vi "Galvos.vi"() -> ()   [LabVIEW 2014]
uses:
  <vilib>/Analysis/1siggen.llb/Ramp Pattern by Samples.vi
  <vilib>/Analysis/NI_AALBase.lvlib
panel:
  in  "Relax":dbl=10.0 format="%0.2p"
  in  "FOV /V":dbl=10.0 format="%0.2p"
  in  "Samples /s":dbl=10.0 format="%0.2p"
  in  "Exposure":dbl=10.0 format="%0.2p"
  out "XY Galvo":dbl[](graph)
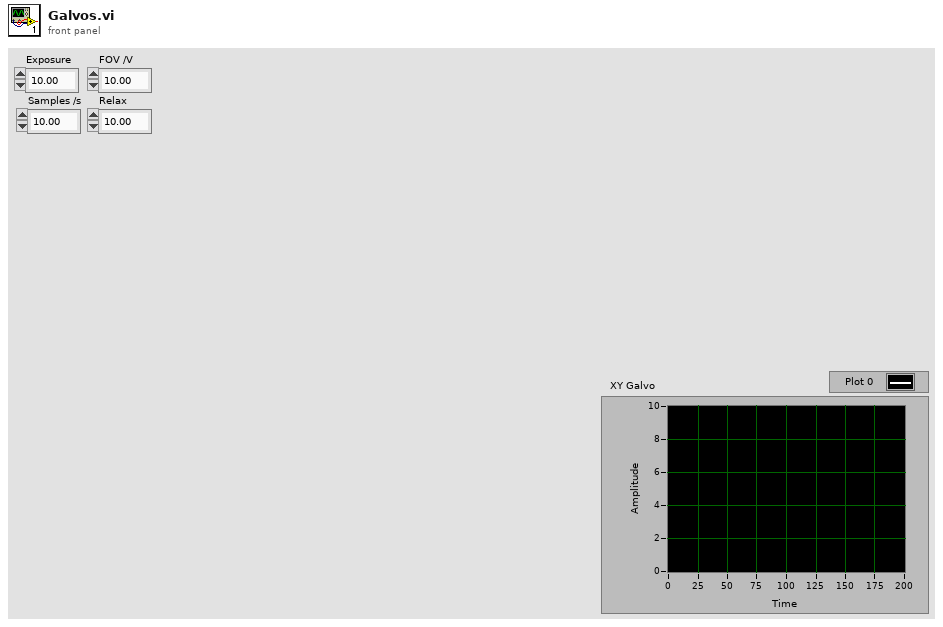
[diagram p1: front panel]
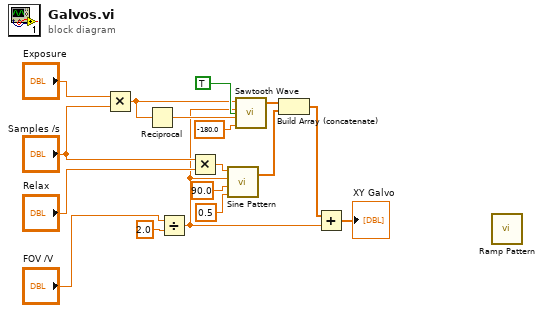
[diagram p0: block diagram]
diagram:
  n1 = Multiply(x="Exposure", y="Samples /s") -> (x*y=w10:dbl)
  n2 = Reciprocal(x=w10) -> (1/x=w12:dbl)
  n3 = Divide(x="FOV /V", y=2.0) -> (x/y=w1:dbl)
  n4 = Multiply(x="Samples /s", y="Relax") -> (x*y=w2:dbl)
  n5 = call <vilib>:"Sine Pattern.vi"("cycles"=0.5, "phase(degrees)"=90.0, "amplitude"=w1, "samples"=w2) -> ("Sinusoidal Pattern"=w14:dbl[])  [unwired: 1 out]
  n6 = call <vilib>:"Sawtooth Wave.vi"("samples"=w10, "amplitude"=w1, "frequency"=w12, "phase in"=-180.0, "reset phase"=TRUE) -> ("sawtooth wave"=w13:dbl[])  [unwired: 2 out]
  n7 = Build Array (concatenate)(w13, w14) -> (w8:dbl[])
  n8 = Add(x=w8, y=w1) -> (x+y=→"XY Galvo":dbl[])
  n9 = call-poly <vilib>:"Ramp Pattern.vi"() -> ()  [unwired: 10 in, 2 out]
